vi "Reef Align Play Path.vi"(4 "PID setpoint":dbl, 6 "Tag ID":dbl, 7 "PID Constants":T1, 8 "Operation":T2, 9 "Auto Data":T14, 10 "Motors":T3 {"Radii (ft)"."Right Back Position" format="%.2f"; "Radii (ft)"."Right Front Position" format="%.2f"; "Radii (ft)"."Left Back Position" format="%.2f"; "Radii (ft)"."Left Front Position" format="%.2f"; "Pigeon2"."Type" items=["CAN"=352321536, "TalonSRX"=33554432]}, 11 "AprilTag Offset":dbl) -> (0 "Auto Done?":bool)   [LabVIEW 2023]
uses:
  swerve/Type Definitions/Data/Robot Velocities.ctl
  swerve/Type Definitions/Hardware/Swerve Drives/(NEO-NEO-ThroughBore-Pigeon2) Swerve.ctl
  swerve/Type Definitions/Hardware/4 Motor Sets/(NEO & NEO 550) 4 Motor Set.ctl
  <vilib>/Rock Robotics/WPI/MotorControl/WPI_MotorControlDeviceRef.ctl
  <vilib>/Rock Robotics/WPI/MotorControl/WPI_MotorControlType.ctl
  <vilib>/Rock Robotics/SystemInterfaces/DIO/FPGA_DIOPWMChannel.ctl
  <vilib>/Rock Robotics/WPI/PWM/WPI_PWMDeadband.ctl
  <vilib>/Rock Robotics/SystemInterfaces/DIO/FPGA_DIOChannel.ctl
  <vilib>/Rock Robotics/WPI/ThirdParty/Phoenix-LabVIEW/Pigeon IMU/CTRE_PigeonIMU_DeviceRef.ctl
  <vilib>/Rock Robotics/WPI/ThirdParty/Phoenix-LabVIEW/Pigeon IMU/CTRE_PigeonIMU_ConnectionType.ctl
  swerve/Type Definitions/Data/Pod Positions.ctl
  Implementation/Drive Operations.ctl
  <vilib>/Platform/TimedLoop/XDataNode/timing_clust.ctl
  <vilib>/Platform/TimedLoop/XDataNode/nitl_modes.ctl
  <vilib>/Platform/TimedLoop/XDataNode/wakeup.ctl
  <vilib>/Rock Robotics/WPI/ThirdParty/REV Robotics/REVLib/Typedef/Spark MAX Control Type.ctl
  <vilib>/Rock Robotics/WPI/DriverStation/WPI_DriverStationRobotMode2.ctl
  c1434f1d-cc94-402a-bfa5-996335562ac8.vi
  Framework/Robot Global Data.vi
  <vilib>/Rock Robotics/WPI/ThirdParty/REV Robotics/REVLib/SubVI/Public/SPARK Get Device Status Output Current.vi
  <vilib>/Platform/TimedLoop/XDataNode/XDataNode.xnode
  <vilib>/Platform/TimedLoop/XDataNode/XDNodeRunTimeDep.lvlib
panel:
  in  "Aligned Threshold":dbl=25.0
  out "Output Current":dbl(graph)
  in  "Int per ft":dbl=0.75
  # "describes what the angle of the tag is (determined in Drive Controller)"
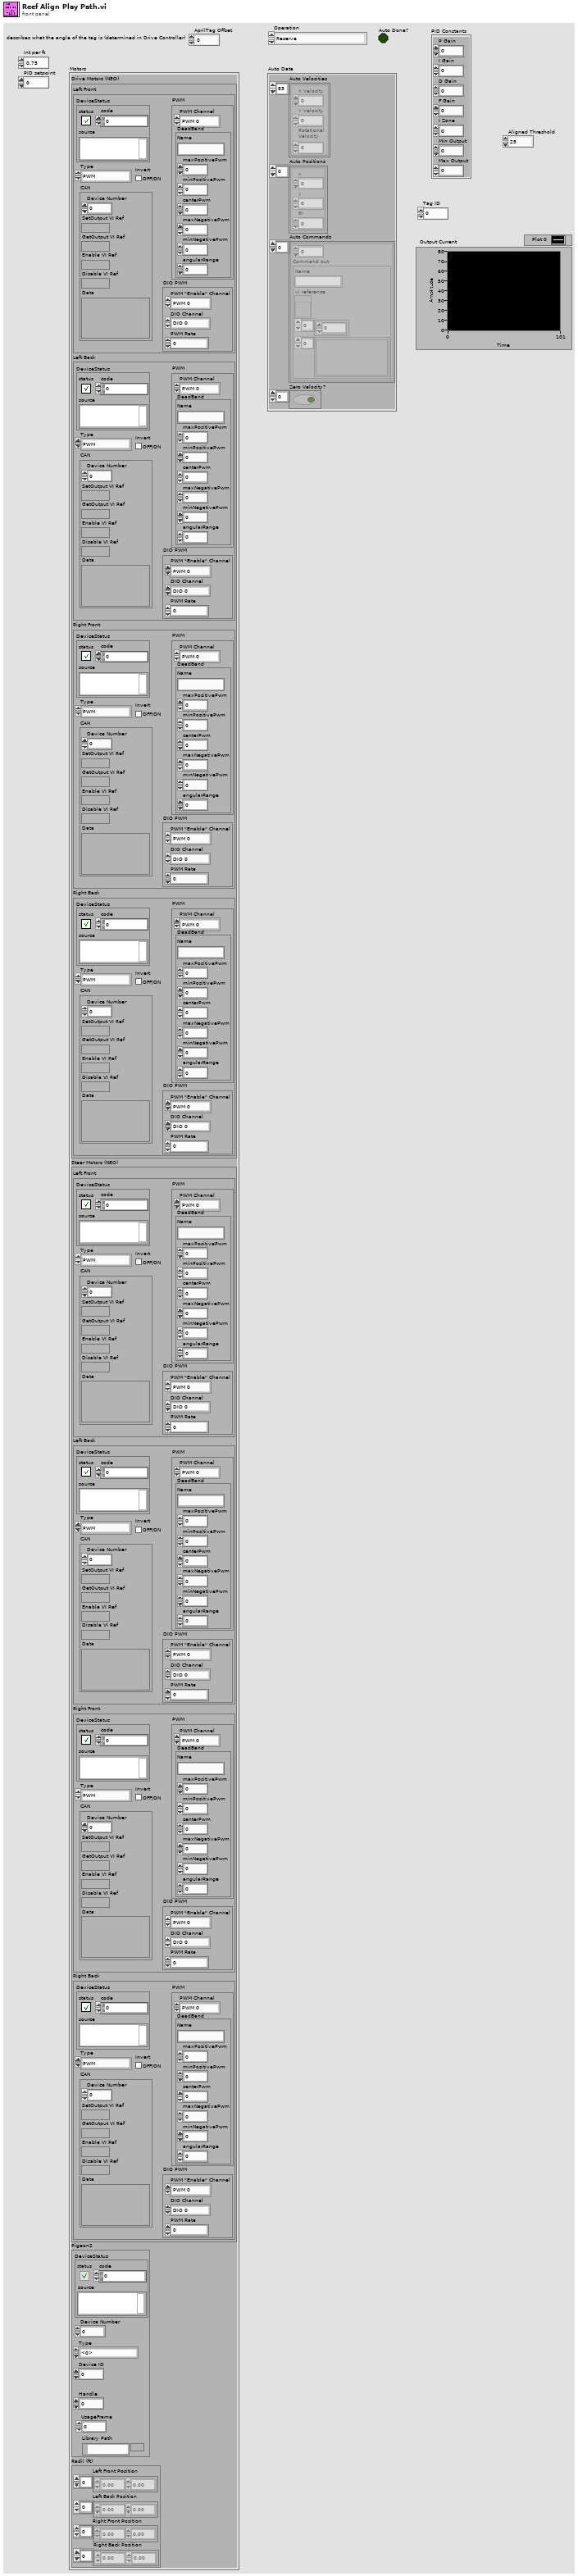
[diagram p1: front panel]
types:
  T1 = cluster{"P Gain":dbl, "I Gain":dbl, "D Gain":dbl, "F Gain":dbl, "I Zone":dbl, "Min Output":dbl, "Max Output":dbl}
  T2 = typedef "Drive Operations.ctl" = enum16{"Reserve", "Read Current", "Immediate", "Calibrate", "Reef Align", "Auto"}
  T3 = typedef "(NEO-NEO-ThroughBore-Pigeon2) Swerve.ctl" = cluster{"Drive Motors (NEO)":T4, "Steer Motors (NEO)":T4, "Pigeon2":T10, "Radii (ft)":T12}
  T4 = typedef "(NEO & NEO 550) 4 Motor Set.ctl" = cluster{"Left Front":T5, "Left Back":T5, "Right Front":T5, "Right Back":T5}
  T5 = typedef "WPI_MotorControlDeviceRef.ctl" = cluster{"DeviceStatus":errorcluster, "Type":T6, "PWM":cluster{"PWM Channel":T7, "DeadBand":T8}, "CAN":cluster{"Device Number":u8, "SetOutput VI Ref":variant, "GetOutput VI Ref":variant, "Enable VI Ref":variant, "Disable VI Ref":variant, "Data":variant}, "Invert":bool, "DIO PWM":cluster{"PWM \"Enable\" Channel":T7, "DIOChannel":T9, "PWM Rate":dbl}}
  T6 = typedef "WPI_MotorControlType.ctl" = enum16{"PWM", "CAN", "DIO PWM"}
  T7 = typedef "FPGA_DIOPWMChannel.ctl" = enum8{"PWM 0", "PWM 1", "PWM 2", "PWM 3", "PWM 4", "PWM 5", "PWM 6", "PWM 7", "PWM 8", "PWM 9", "PWM MXP 0", "PWM MXP 1", "PWM MXP 2", "PWM MXP 3", "PWM MXP 4", "PWM MXP 5", "PWM MXP 6", "PWM MXP 7", "PWM MXP 8", "PWM MXP 9", "Invalid"}
  T8 = typedef "WPI_PWMDeadband.ctl" = cluster{"Name":string, "maxPositivePwm":i32, "minPositivePwm":i32, "centerPwm":i32, "maxNegativePwm":i32, "minNegativePwm":i32, "angularRange":u16}
  T9 = typedef "FPGA_DIOChannel.ctl" = enum8{"DIO 0", "DIO 1", "DIO 2", "DIO 3", "DIO 4", "DIO 5", "DIO 6", "DIO 7", "DIO 8", "DIO 9", "DIO MXP 0", "DIO MXP 1", "DIO MXP 2", "DIO MXP 3", "DIO MXP 4", "DIO MXP 5", "DIO MXP 6", "DIO MXP 7", "DIO MXP 8", "DIO MXP 9", "DIO MXP 10", "DIO MXP 11", "DIO MXP 12", "DIO MXP 13", "DIO MXP 14", "DIO MXP 15", "SPI Port CS1", "SPI Port CS2", "SPI Port CS3", "SPI Port MISO", "SPI Port MOSI", "Invalid"}
  T10 = typedef "CTRE_PigeonIMU_DeviceRef.ctl" = cluster{"DeviceStatus":errorcluster, "Device Number":u8, "Type":T11, "Device ID":u32, "Handle":u64, "UsageFrame":u32, "Library Path":path}
  T11 = typedef "CTRE_PigeonIMU_ConnectionType.ctl" = u32
  T12 = typedef "Pod Positions.ctl" = cluster{"Left Front Position":dbl[], "Left Back Position":dbl[], "Right Front Position":dbl[], "Right Back Position":dbl[]}
  T13 = typedef "Robot Velocities.ctl" = cluster{"X Velocity":dbl, "Y Velocity":dbl, "Rotational \nVelocity":dbl}
  T14 = cluster{"Auto Velocities":T13[], "Auto Positions":cluster{"x":dbl, "y":dbl, "th":dbl}[], "Auto Commands":cluster{dbl, "Command out":cluster{"Name":string, "vi reference":refnum<vi>, i32[], variant[]}}[], "Zero Velocity?":bool[]}
  T15 = cluster{"Time (s)":dbl, "Command out":cluster{"Name":string, "vi reference":refnum<vi>, i32[], variant[]}}
  T16 = typedef "Spark MAX Control Type.ctl" = enum16{"Percent VBus", "Voltage", "Velocity", "Position", "Smart Motion", "Current", "Smart Velocity", "MAXMotion Position", "MAXMotion Velocity"}
  T17 = cluster{"Left Front":dbl, "Left Back":dbl, "Right Front":dbl, "Right Back":dbl}
  T18 = typedef "XDNodeRunTimeDep.lvlib/timing_clust.ctl" = cluster{"Expected End [f-1]":u64, "Actual End [f-1]":u64, "Finished Late? [f-1]":bool, "Expected End [i-1]":u64, "Actual End [i-1]":u64, "Finished Late? [i-1]":bool, "Expected Start [i]":u64, "Actual Start [i]":u64, "Expected Start [f]":u64, "Actual Start [f]":u64, "Source Name":string, "Structure Name":string, "Period":i64, "Deadline":i64, "Offset":i64, "Start":i64, "Priority":i32, "Timeout":i32, "Mode":T19, "Wakeup Reason":T20, "Error":errorcluster, "Source Type":string, "Secondary Source Type":string, "Global End Time":u64, "Global Start Time":u64, "Frame Duration":u64, "Iteration Duration":u64, "Assigned CPU":i32, "I/O Scan Engine Mode":u32}
  T19 = typedef "XDNodeRunTimeDep.lvlib/nitl_modes.ctl" = enum32{"No Change", "Process missed periods, maintain original phase", "Discard missed periods, maintain original phase", "Process missed periods, ignore original phase", "Discard missed periods, ignore original phase"}
  T20 = typedef "XDNodeRunTimeDep.lvlib/wakeup.ctl" = enum32{"Normal", "Aborted", "Asynchronous wakeup", "Timing source error", "Timed loop error", "Timeout"}
  T21 = cluster{dbl, "Command out":cluster{"Name":string, "vi reference":refnum<vi>, i32[], variant[]}}[]
  T22 = cluster{"Field Centric":bool, "Reef Centric":bool}
  T23 = typedef "WPI_DriverStationRobotMode2.ctl" = enum16{"Autonomous Disabled", "Autonomous Enabled", "Teleop Disabled", "Teleop Enabled", "Disconnected", "Finish", "Test Disabled", "Test Enabled", "Emergency Stopped"}
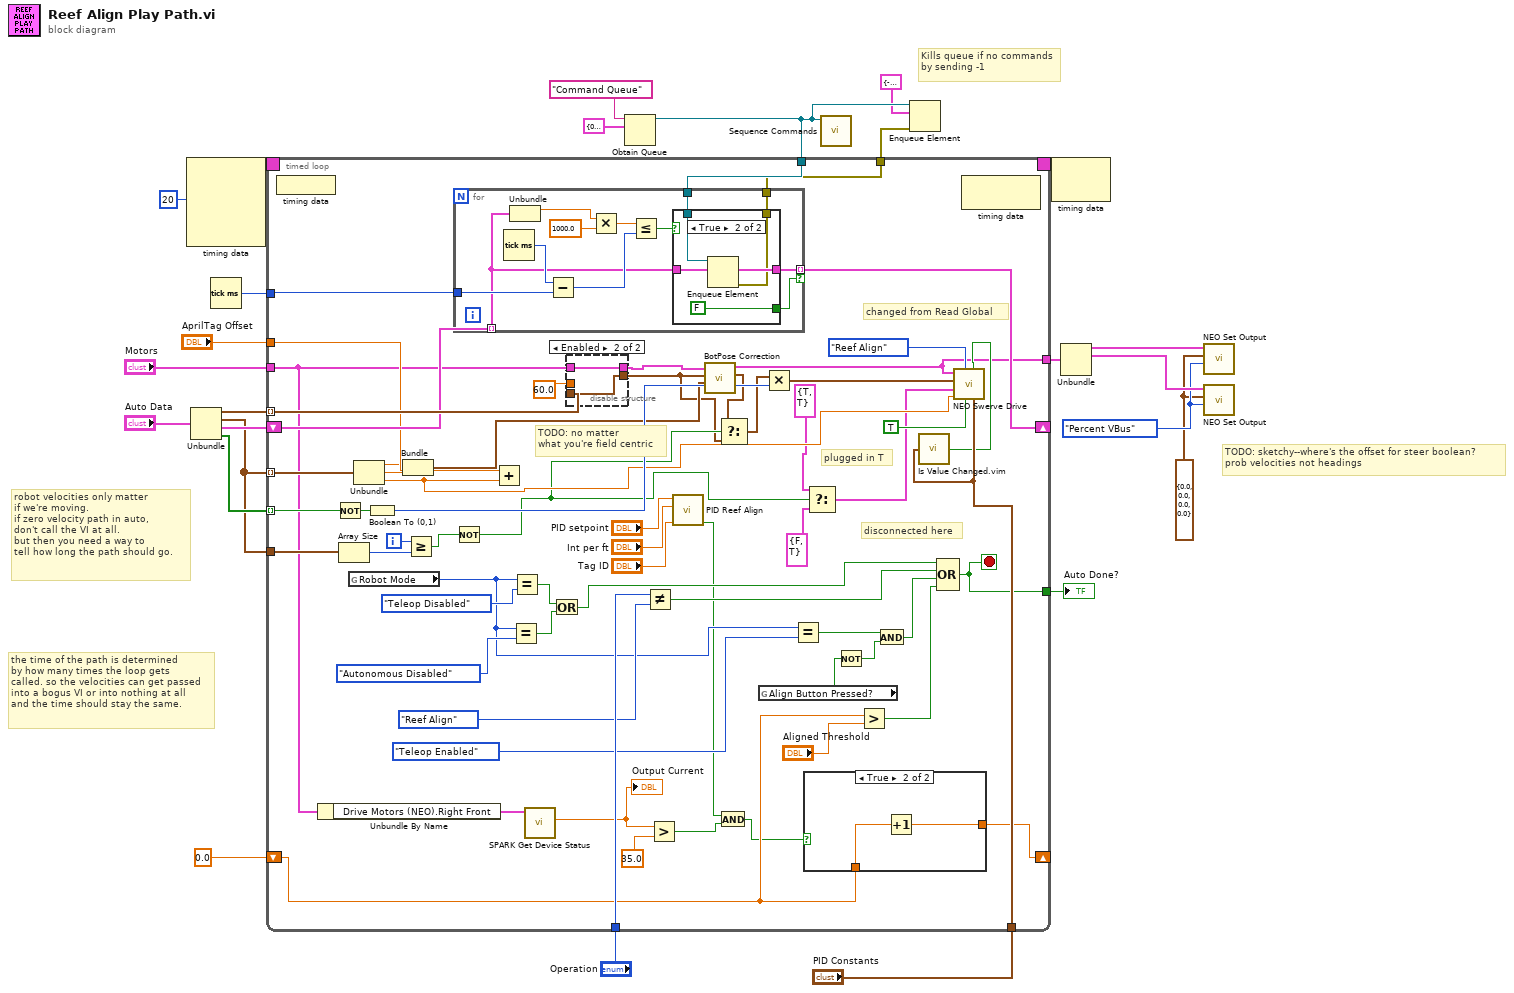
[diagram p0: block diagram]
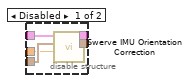
[diagram p2: hidden frame]
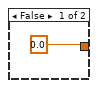
[diagram p3: hidden frame]
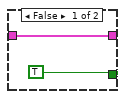
[diagram p4: hidden frame]
diagram:
  w10 = Spark_MAX_Control_Type."Percent VBus" ("Control Mode")
  w9 = T17 {"Left Front"=0.0, "Left Back"=0.0, "Right Front"=0.0, "Right Back"=0.0} ("Setpoints")
  # "the time of the path is determined\nby how many times the loop gets\ncalled. so the velocities can get passed\ninto a bogus VI or into nothing at all\nand the time should stay the same."
  # "robot velocities only matter\nif we're moving.\nif zero velocity path in auto,\ndon't call the VI at all.\nbut then you need a way to \ntell how long the path should go."
  # "TODO: sketchy--where's the offset for steer boolean?\nprob velocities not headings"
  # "Kills queue if no commands by sending -1"
  n1 = node-c288(i64 20 ("Period")) -> (w25:T18)  [unwired: 3 in]
  n2 = Unbundle("Auto Data") -> ("Auto Velocities"=w18:T13[], "Auto Positions"=w19:cluster{"x":dbl, "y":dbl, "th":dbl}[], "Auto Commands"=w21:T21, "Zero Velocity?"=w22:bool[])
  n3 = Tick Count (ms)() -> (millisecond timer value=w20:u32)
  n4 = Obtain Queue(name (unnamed)="Command Queue", element data type=T15 {"Time (s)"=0.0, "Command out"={"Name"="", "vi reference"=refnum, [], []}} ("element")) -> (queue out=w6:refnum<queue>)  [unwired: 3 in, 2 out]
  n5 = timed-loop {
    timing: w25 -> [_]
    timing-out: [_] -> w24
    tunnel: "Motors" -> [w47]
    tunnel: [w35] -> w8
    tunnel: w18 -> [w86] mode=indexing
    tunnel: w19 -> [w85] mode=indexing
    tunnel: w19 -> [w55]
    tunnel: w20 -> [w84]
    tunnel: w6 -> [w83]
    shift-right: [w81] -> _
    shift-left: w21 -> [w80]
    tunnel: w22 -> [w76] mode=indexing
    tunnel: [w69] -> w23
    tunnel: "Operation" -> [w75]
    tunnel: [w74] -> w5
    tunnel: "PID Constants" -> [w73]
    tunnel: "AprilTag Offset" -> [w67]
    shift-right: [w45] -> _
    shift-left: 0.0 -> [w44]
    i -> [w87]
    stop <- w69 stop-if-true
    # "TODO: no matter\nwhat you're field centric"
    # "changed from Read Global"
    # "plugged in T"
    # "disconnected here"
    n6 = node-c288() -> ()  [unwired: 1 in]
    n7 = Unbundle By Name(w47) -> ("Drive Motors (NEO).Right Front"=w46:T5)
    n8 = Not(x=w76) -> (.not. x?=w79:bool)
    n9 = Array Size(array=w55) -> (size(s)=w88:i32)
    n10 = global read "Robot Global Data.vi" "Robot Mode"() -> (w60:T23)
    n11 = Unbundle(w85) -> ("x"=w34:dbl, "y"=w33:dbl, "th"=w66:dbl)
    n12 = Boolean To (0,1)(Boolean=w79) -> (0, 1=w78:i16)
    n13 = Bundle("x"=w34, "y"=w33) -> (w32:cluster{"x":dbl, "y":dbl})  [unwired: 1 in]
    n14 = Greater Or Equal?(x=w87, y=w88) -> (x >= y?=w49:bool)
    n15 = for {
      tunnel: w84 -> [w109]
      tunnel: w83 -> [w103]
      tunnel: w80 -> [w100] mode=indexing
      tunnel: [w102] -> w81 mode=indexing if=w101
      tunnel: [w99] -> w74
      n16 = Tick Count (ms)() -> (millisecond timer value=w110:u32)
      n17 = Unbundle(w100) -> (w108:dbl)  [unwired: 1 out]
      n18 = Subtract(x=w110, y=w109) -> (x-y=w105:u32)
      n19 = Multiply(x=w108, y=1000.0) -> (x*y=w106:dbl)
      n20 = Less Or Equal?(x=w106, y=w105) -> (x <= y?=w104:bool)
      n21 = case shown="True" w104 {
        tunnel: w103 -> [_ w116]
        tunnel: w100 -> [w111 w115]
        tunnel: [w111 w115] -> w102
        tunnel: [TRUE FALSE] -> w101
        tunnel: [_ w113] -> w99
        frame False {
        }
        frame True {
          n22 = Enqueue Element(queue=w116, element=w115) -> (error out=w113:errorcluster)  [unwired: 2 in, 2 out]
        }
      }
    }
    n23 = Not(x=w49) -> (.not. x?=w28:bool)
    n24 = Add(x=w67, y=w66) -> ()  [unwired: 1 out]
    n25 = Equal?(x=w60, y=WPI_DriverStationRobotMode2."Autonomous Disabled") -> (x = y?=w64:bool)
    n26 = Equal?(x=w60, y=WPI_DriverStationRobotMode2."Teleop Disabled") -> (x = y?=w63:bool)
    n27 = call-poly <vilib>:"SPARK Get Device Status.vi"("MotorControlDevRef in"=w46) -> ("Current"=w40:dbl)  [unwired: 7 in, 3 out]
    "Output Current" <- w40
    n28 = Or(x=w63, y=w64) -> (x .or. y?=w62:bool)
    n29 = disable-structure shown="Enabled" {
      disable-tunnel: w86 -> [w93 w94]
      disable-tunnel: w47 -> [w92 w95]
      disable-tunnel: [w91 w95] -> w36
      disable-tunnel: [w90 w94] -> w26
      disable-tunnel: 60.0 ("Setpoint") -> [w89 _]
      frame Disabled {
        n30 = call "Swerve IMU Orientation Correction.vi"("Setpoint"=w89, "Robot Velocities In"=w93, "Motors In"=w92) -> ("Robot Velocities Out"=w90:T13, "Motors Out"=w91:T3)  [unwired: 7 in]
      }
      frame Enabled {
      }
    }
    n31 = Not Equal?(x=w75, y=Drive_Operations."Reef Align") -> (x != y?=w77:bool)
    n32 = Greater?(x=w40, y=35.0) -> (0:w38:bool)
    n33 = call "PID Reef Align.vi"("Tag ID"="Tag ID", "Int per ft"="Int per ft", "setpoint"="PID setpoint") -> ("PID Happy?"=w41:bool)  [unwired: 5 in, 1 out]
    n34 = call "BotPose Correction.vi"("Pos In"=w32, "Robot Velocities In"=w26, "Motors In"=w36) -> ("Robot Velocities Out"=w27:T13, "Motors Out"=w35:T3)  [unwired: 7 in]
    n35 = And(x=w41, y=w38) -> (x .and. y?=w42:bool)
    n36 = Select(t=w27, s=w28, f=w26) -> (s? t:f=w29:T13)
    n37 = global read "Robot Global Data.vi" "Align Button Pressed?"() -> (w65:bool)
    n38 = Multiply(x=w29, y=w78) -> (x*y=w31:T13)
    n39 = Equal?(x=w60, y=WPI_DriverStationRobotMode2."Teleop Enabled") -> (x = y?=w58:bool)
    n40 = case shown="True" w42 {
      tunnel: w44 -> [_ w98]
      tunnel: [0.0 w97] -> w45
      frame False {
      }
      frame True {
        n41 = Increment(x=w98) -> (x+1=w97:dbl)
      }
    }
    n42 = Select(t=T22 {"Field Centric"=TRUE, "Reef Centric"=TRUE} ("Drive Conditions"), s=w28, f=T22 {"Field Centric"=FALSE, "Reef Centric"=TRUE}) -> (s? t:f=w48:T22)
    n43 = Not(x=w65) -> (.not. x?=w57:bool)
    n44 = Greater?(x=w44, y="Aligned Threshold") -> (0:w37:bool)
    n45 = And(x=w58, y=w57) -> (x .and. y?=w56:bool)
    n46 = call "Is Value Changed.vim"("value"=w73) -> ("changed or first call?"=w72:bool)
    n47 = Compound Arithmetic op=OR(w62, w77, w56, w37) -> (w69:bool)
    n48 = call "NEO Swerve Drive.vi"("PID Constants"=w73, "Configure?"=w72, "Angle Align"=TRUE, "Operation"=Drive_Operations."Reef Align", "Offset from 0"=w66, "Drive Conditions"=w48, "Robot Velocities"=w31, "Swerve Drive"=w35) -> ()  [unwired: 3 in, 1 out]
    n49 = node-c288() -> ()  [unwired: 1 in, 1 out]
  }
  "Auto Done?" <- w23
  n50 = call "Sequence Commands.vi"("queue in"=w6) -> ()  [unwired: 11 in]
  n51 = Enqueue Element(queue=w6, element=T15 {"Time (s)"=-1.0, "Command out"={"Name"="", "vi reference"=refnum, [], []}}, error in (no error)=w5) -> ()  [unwired: 1 in, 3 out]
  n52 = node-c288(w24) -> ()  [unwired: 1 out]
  n53 = Unbundle(w8) -> ("Drive Motors (NEO)"=w12:T4, "Steer Motors (NEO)"=w11:T4)  [unwired: 2 out]
  n54 = call "NEO Set Output.vi"("Control Mode"=w10, "Setpoints"=w9, "Motors"=w12) -> ()  [unwired: 9 in]
  n55 = call "NEO Set Output.vi"("Control Mode"=w10, "Setpoints"=w9, "Motors"=w11) -> ()  [unwired: 9 in]
